vi "Unflatten.vi"(8 "error in (no error)":errorcluster, 11 "Analog Out Scan in":refnum<class "Analog Output Scan.lvclass">) -> (0 "error out":errorcluster, 3 "Analog Out Scan out":refnum<class "Analog Output Scan.lvclass">)   [LabVIEW 2017, in "Analog Output Scan.lvclass"]
uses:
  Analog Output Scan.lvclass
  Analog Output Scan.lvclass/Analog Output Scan.ctl
  Global/File Locations.vi
  Scanner/Scanner.lvclass
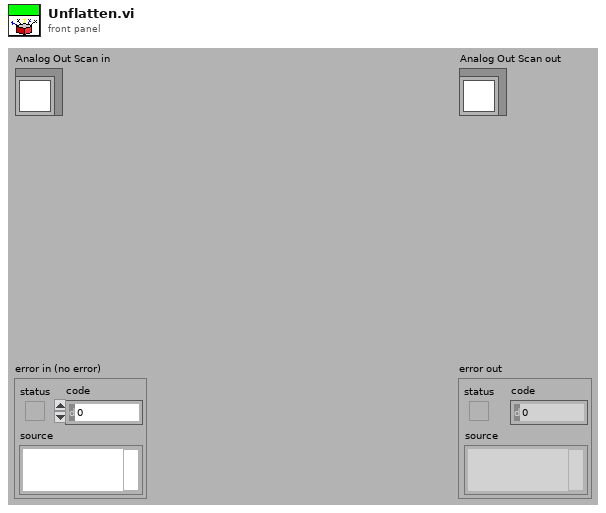
[diagram p1: front panel]
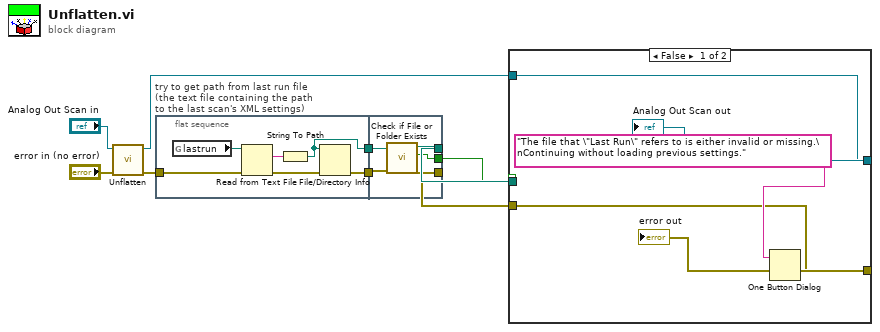
[diagram p0: block diagram]
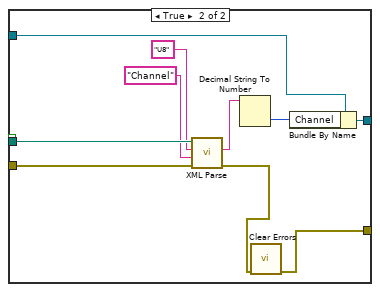
[diagram p2: hidden frame]
diagram:
  n1 = call-parent "Unflatten.vi"("error in (no error)"="error in (no error)", "Scanner in"="Analog Out Scan in") -> ("error out"=w8:errorcluster, "Scanner out"=w11:refnum<class "Analog Output Scan.lvclass">)  [unwired: 8 in]
  n2 = flat-sequence "try to get path from last run file\n(the text file containing the path\nto the last scan's XML settings)" {
    tunnel: w8 -> [w12]
    tunnel: [w17] -> w3
    tunnel: [w13] -> w2
    tunnel: [w21] -> w5
    tunnel: [w22] -> w6
    tunnel: w3 -> [w19]
    tunnel: w2 -> [w20]
    tunnel: [w18] -> w1
    frame #0 {
      n3 = global read "File Locations.vi" "lastrun"() -> (w15:path)
      n4 = Read from Text File(file (use dialog)=w15, error in=w12) -> (text=w16:string, error out=w14:errorcluster)  [unwired: 4 out]
      n5 = String To Path(string=w16) -> (path=w17:path)
      n6 = File/Directory Info(path=w17, error in=w14) -> (error out=w13:errorcluster)  [unwired: 6 out]
    }
    frame #1 {
      n7 = call <vilib>:"Check if File or Folder Exists.vi"("error in (no error)"=w20, "path"=w19) -> ("error out"=w21:errorcluster, "file or folder exists?"=w18:bool, "dup path"=w22:path)  [unwired: 7 in]
    }
  }
  n8 = case shown="False" w1 {
    tunnel: w11 -> [w23 w35]
    tunnel: [w23 w34] -> w7
    tunnel: w6 -> [_ w33]
    tunnel: w5 -> [w24 w30]
    tunnel: [w24 w27] -> w4
    frame False {
      n9 = One Button Dialog(message="The file that \"Last Run\" refers to is either invalid or missing.\nContinuing without loading previous settings.") -> ()  [unwired: 1 in, 1 out]
    }
    frame True {
      n10 = call "XML Parse.vi"("error in (no error)"=w30, "Name String"="Channel", "Type String"="U8", "Path"=w33) -> ("error out"=w26:errorcluster, "String Out"=w29:string)  [unwired: 6 in]
      n11 = Decimal String To Number(string=w29) -> (number=w28:i32)  [unwired: 2 in, 1 out]
      n12 = call <vilib>:"Clear Errors.vi"("error in (no error)"=w26) -> ("error out"=w27:errorcluster)  [unwired: 5 in, 1 out]
      n13 = Bundle By Name(cluster=w35, "Channel"=w28) -> (w34:refnum<class "Analog Output Scan.lvclass">)
    }
  }
  "error out" <- w4
  "Analog Out Scan out" <- w7
